vi "ROI entry- extract anc check ROI data.vi"(8 "error in (no error)":errorcluster, 10 "ROI File data":dbl[][](array[numeric]), 11 "Old ROI file path":path) -> (0 "error out":errorcluster, 1 "Latest AOL Z values":dbl[](array[numeric]), 2 "Last ROI Enum":T1, 3 "Array":T2[](array[typedef]) {"Zoom" min=1.0 max=10.0 step=0.10000000149011612}, 5 "ROI type consistent":bool)   [LabVIEW 2017]
uses:
  Typedefs/ROI spec.ctl
  Typedefs/ROI ID Enum.ctl
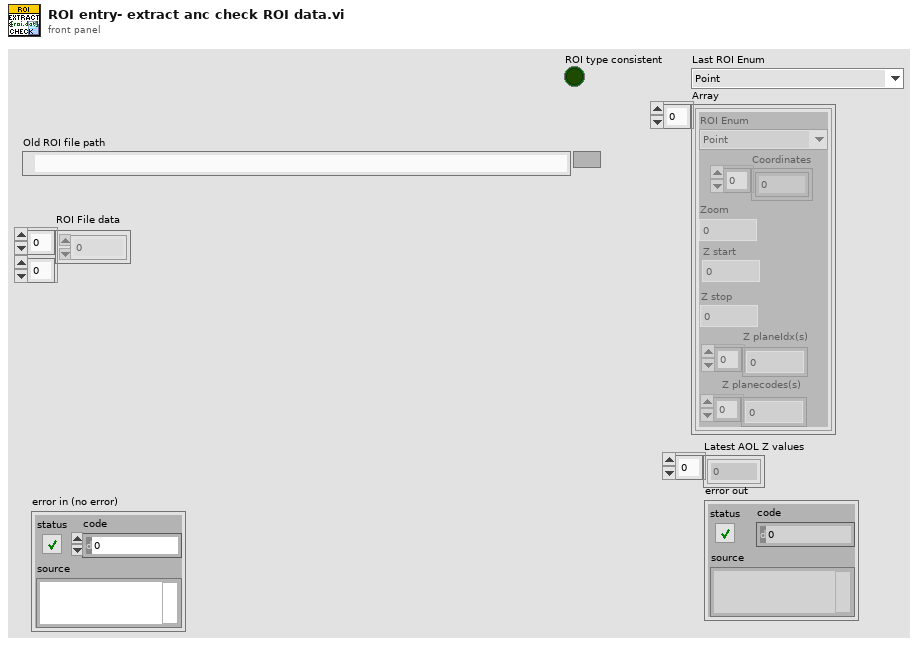
[diagram p1: front panel]
types:
  T1 = typedef "ROI ID Enum.ctl" = enum16{"Point", "MiniScan", "Comp. MiniScan", "Rectangle", "Comp. volume", "Arb. plane point"}
  T2 = typedef "ROI spec.ctl" = cluster{"Coordinates":i32[], "Zoom":dbl, "ROI Enum":T1, "Z planeIdx(s)":i32[], "Z planecodes(s)":u8[], "Z start":dbl, "Z stop":dbl}
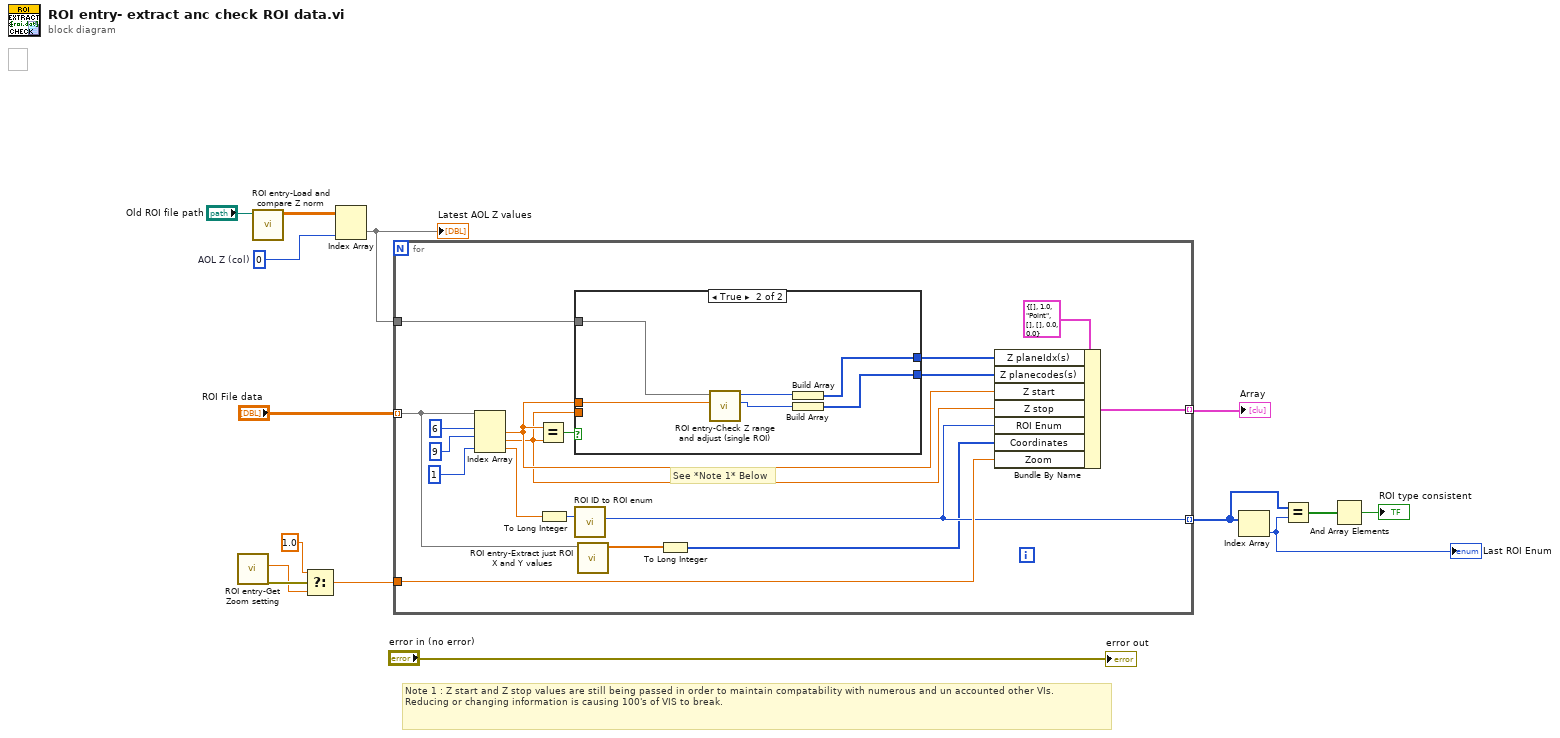
[diagram p0: block diagram]
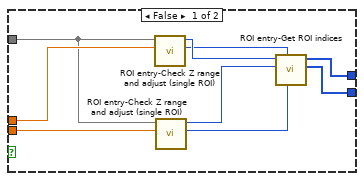
[diagram p2: hidden frame]
diagram:
  w13 = 0  # AOL Z (col)
  # "Note 1 : Z start and Z stop values are still being passed in order to maintain compatability with numerous and un accounted other VIs. \nReducing or changing information is causing 100's of VIS to break."
  n1 = call "ROI entry-Get Zoom setting.vi"() -> ("error out"=w11:errorcluster, "Zoom Value"=w10:dbl)  [unwired: 9 in, 1 out]
  n2 = call "ROI entry-Load and compare Z norm.vi"("Old ROI file path"="Old ROI file path") -> ("Latest Zplane_Pockels_Values file data (header removed)"=w14:dbl[][])  [unwired: 4 in, 6 out]
  n3 = Select(t=1.0, s=w11, f=w10) -> (s? t:f=w8:dbl)
  n4 = Index Array(array=w14, index (col)=w13) -> (element=w6:dbl[])  [unwired: 1 in]
  "Latest AOL Z values" <- w6
  n5 = for {
    tunnel: "ROI File data" -> [w28] mode=indexing
    tunnel: w8 -> [w25]
    tunnel: [w24] -> w7 mode=indexing
    tunnel: w6 -> [w23]
    tunnel: [w20] -> w5 mode=indexing
    # "See *Note 1* Below"
    n6 = Index Array(array=w28, index #1=6, index #2=9, index #3=1 ("index")) -> (element #1=w17:dbl, element #2=w16:dbl, element #3=w26:dbl)
    n7 = Equal?(x=w17, y=w16) -> (x = y?=w30:bool)
    n8 = To Long Integer(number=w26) -> (32bit integer=w27:i32)
    n9 = case shown="True" w30 {
      tunnel: w17 -> [w42 w47]
      tunnel: w16 -> [w40 _]
      tunnel: w23 -> [w41 w48]
      tunnel: [w35 w45] -> w22
      tunnel: [w34 w43] -> w21
      frame False {
        n10 = call "ROI entry-Check Z range and adjust (single ROI).vi"("AOL Z plane value"=w42, "Latest Zplane_Pockels_Values file data (header removed)"=w41) -> ("Z plane code"=w38:u8, "Z plane Index"=w39:i32)  [unwired: 7 in, 1 out]
        n11 = call "ROI entry-Check Z range and adjust (single ROI).vi"("AOL Z plane value"=w40, "Latest Zplane_Pockels_Values file data (header removed)"=w41) -> ("Z plane code"=w36:u8, "Z plane Index"=w37:i32)  [unwired: 7 in, 1 out]
        n12 = call "ROI entry-Get ROI indices.vi"("Z stop code"=w36, "Z start code"=w38, "Z stop index"=w37, "Z start Index"=w39) -> ("Z codes"=w34:u8[], "Z Idx(s)"=w35:i32[])  [unwired: 6 in]
      }
      frame True {
        n13 = call "ROI entry-Check Z range and adjust (single ROI).vi"("AOL Z plane value"=w47, "Latest Zplane_Pockels_Values file data (header removed)"=w48) -> ("Z plane code"=w44:u8, "Z plane Index"=w46:i32)  [unwired: 7 in, 1 out]
        n14 = Build Array(w46) -> (w45:i32[])
        n15 = Build Array(w44) -> (w43:u8[])
      }
    }
    n16 = call "ROI ID to ROI enum.vi"("ROI ID"=w27) -> ("ROI Enum"=w20:T1)  [unwired: 6 in]
    n17 = call "ROI entry-Extract just ROI X and Y values.vi"("Single ROI component data"=w28) -> ("X and Y values array"=w19:dbl[])  [unwired: 10 in]
    n18 = To Long Integer(number=w19) -> (32bit integer=w18:i32[])
    n19 = Bundle By Name(cluster=T2 {"Coordinates"=[], "Zoom"=1.0, "ROI Enum"=enum."Point", "Z planeIdx(s)"=[], "Z planecodes(s)"=[], "Z start"=0.0, "Z stop"=0.0} ("input cluster"), "Z planeIdx(s)"=w22, "Z planecodes(s)"=w21, "Z start"=w17, "Z stop"=w16, "ROI Enum"=w20, "Coordinates"=w18, "Zoom"=w25) -> (w24:T2)
  }
  "Array" <- w7
  n20 = Index Array(array=w5) -> (element=w2:T1)  [unwired: 1 in]
  "Last ROI Enum" <- w2
  n21 = Equal?(x=w5, y=w2) -> (x = y?=w4:bool[])
  n22 = And Array Elements(Boolean array=w4) -> (logical AND=→"ROI type consistent":bool)
  "error out" <- "error in (no error)"
